vi "Teleop.vi"(10 "Match Info":T1={"Autonomous Elapsed Seconds"=0.0, "TeleOp Elapsed Seconds"=0.0, "Disabled Elapsed Seconds"=0.0, "Visited Autonomous"=FALSE, "Visited TeleOp"=FALSE, "Visited Disabled"=FALSE, "Autonomous Settings"={"Autonomous Style"=enum."Independent", "VI Refnum"=refnum}}, 11 "Call Context":T2) -> ()   [LabVIEW 2015]
doc: "This VI is called for each TeleOp packet received from the DS where the robot is not disabled. It is often used to read from the joysticks and update I/O or to update setpoints for timed control loops. It should complete and return within 20 milliseconds or it may miss DS packets."
uses:
  <vilib>/Rock Robotics/WPI/DriverStation/WPI_DriverStationDerivedRobotMode.ctl
  <vilib>/Rock Robotics/WPI/DriverStation/WPI_DriverStationMatch Info.ctl
  <vilib>/Rock Robotics/WPI/Solenoid/WPI_SolenoidValue.ctl
  <vilib>/Rock Robotics/WPI/Utilities/WPI_GetSetVariantRefNum.vi
  <vilib>/Rock Robotics/Network Tables/NT Write Boolean Array.vi
  <vilib>/Rock Robotics/Network Tables/NT Write Numeric Array.vi
  <vilib>/Rock Robotics/Network Tables/NT Read Boolean.vi
  <vilib>/Rock Robotics/Network Tables/NT Read Number.vi
  <vilib>/Rock Robotics/WPI/Solenoid/WPI_SolenoidSetEnum.vi
  <vilib>/Rock Robotics/Network Tables/NT Write Boolean.vi
  <vilib>/addons/control/pid/NI_PID_pid.lvlib
  <vilib>/addons/control/pid/pid.llb/PID (DBL).vi
panel:
  out "Angle":dbl
  out "Distance":dbl
  out "Sample Slider 0":dbl(slide) scale=0.0..5.0
  out "Sample Boolean 1":bool
  out "Sample Boolean 0":bool
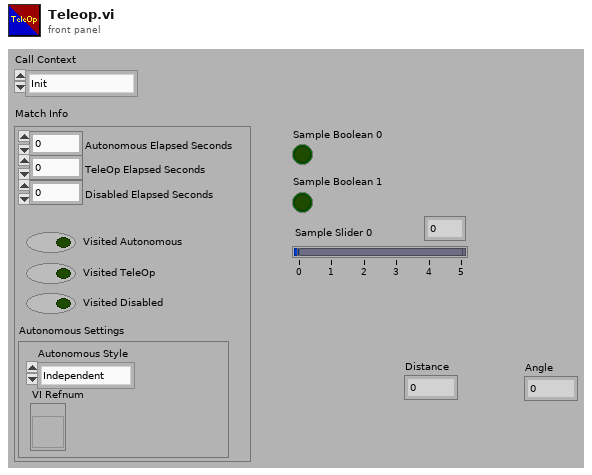
[diagram p1: front panel]
types:
  T1 = typedef "WPI_DriverStationMatch Info.ctl" = cluster{"Autonomous Elapsed Seconds":dbl, "TeleOp Elapsed Seconds":dbl, "Disabled Elapsed Seconds":dbl, "Visited Autonomous":bool, "Visited TeleOp":bool, "Visited Disabled":bool, "Autonomous Settings":cluster{"Autonomous Style":enum16{"Iterative", "Independent"}, "VI Refnum":refnum<vi>}}
  T2 = typedef "WPI_DriverStationDerivedRobotMode.ctl" = enum16{"Init", "Execute", "Stop"}
  T3 = typedef "WPI_SolenoidValue.ctl" = enum16{"Off", "On", "Forward", "Reverse"}
  T4 = typedef "WPI_AnalogChannelDevRef.ctl" = cluster{"DevStatus":errorcluster, "Analog Channel":T5}
  T5 = typedef "FPGA_AIChannel.ctl" = enum8{"AI 0", "AI 1", "AI 2", "AI 3", "AI MXP 0", "AI MXP 1", "AI MXP 2", "AI MXP 3", "Invalid"}
  T6 = typedef "WPI_JoystickDevRef.ctl" = cluster{"Device":T7}
  T7 = typedef "WPI_JoystickDeviceEnum.ctl" = enum16{"USB 0", "USB 1", "USB 2", "USB 3", "USB 4", "USB 5"}
  T8 = cluster{"Buttons[0]":bool, "Buttons[1]":bool, "Buttons[2]":bool, "Buttons[3]":bool, "Buttons[4]":bool, "Buttons[5]":bool, "Buttons[6]":bool, "Buttons[7]":bool, "Buttons[8]":bool}
  T9 = typedef "WPI_MotorControlDeviceRef.ctl" = cluster{"DeviceStatus":errorcluster, "Type":T10, "PWM":cluster{"PWM Channel":T11, "DeadBand":T12}, "CAN":cluster{"Device Number":u8, "Control Mode":T13, "Semaphore":T14, "Max Vout":dbl, "TalonSRX Control Mode":T15}, "Invert":bool}
  T10 = typedef "WPI_MotorControlType.ctl" = enum16{"PWM", "CAN", "CANTalonSRX"}
  T11 = typedef "FPGA_DIOPWMChannel.ctl" = enum8{"PWM 0", "PWM 1", "PWM 2", "PWM 3", "PWM 4", "PWM 5", "PWM 6", "PWM 7", "PWM 8", "PWM 9", "PWM MXP 0", "PWM MXP 1", "PWM MXP 2", "PWM MXP 3", "PWM MXP 4", "PWM MXP 5", "PWM MXP 6", "PWM MXP 7", "PWM MXP 8", "PWM MXP 9", "Invalid"}
  T12 = typedef "WPI_PWMDeadband.ctl" = cluster{"Name":string, "maxPositivePwm":i32, "minPositivePwm":i32, "centerPwm":i32, "maxNegativePwm":i32, "minNegativePwm":i32, "angularRange":u16}
  T13 = typedef "WPI_CANJaguar_ControlMode.ctl" = enum8{"Percent VBus", "Current", "Speed", "Position", "Voltage"}
  T14 = typedef "Semaphore RefNum" = refnum<k1>
  T15 = typedef "WPI_CANTalonSRX_APIControlMode.ctl" = enum8{"Percent VBus", "Speed", "Position", "Slave", "Unchanged / Invalid", "Voltage Compensation", "Current", "Motion Profile"}
  T16 = cluster{"proportional gain (Kc)":dbl, "integral time (Ti, min)":dbl, "derivative time (Td, min)":dbl}
  T17 = typedef "WPI_RobotDriveDevRef.ctl" = cluster{"DevStatus":errorcluster, "Motors[]":T9[], "Square Inputs":bool, "Max Output":dbl}
  T18 = typedef "WPI_SolenoidDevRef.ctl" = cluster{"DevStatus":errorcluster, "Pneumatics Control Module":u8, "Forward Solenoid Channel":T19, "Reverse Solenoid Channel":T19}
  T19 = typedef "WPI_SolenoidChannel.ctl" = enum8{"Solenoid 0", "Solenoid 1", "Solenoid 2", "Solenoid 3", "Solenoid 4", "Solenoid 5", "Solenoid 6", "Solenoid 7", "Invalid"}
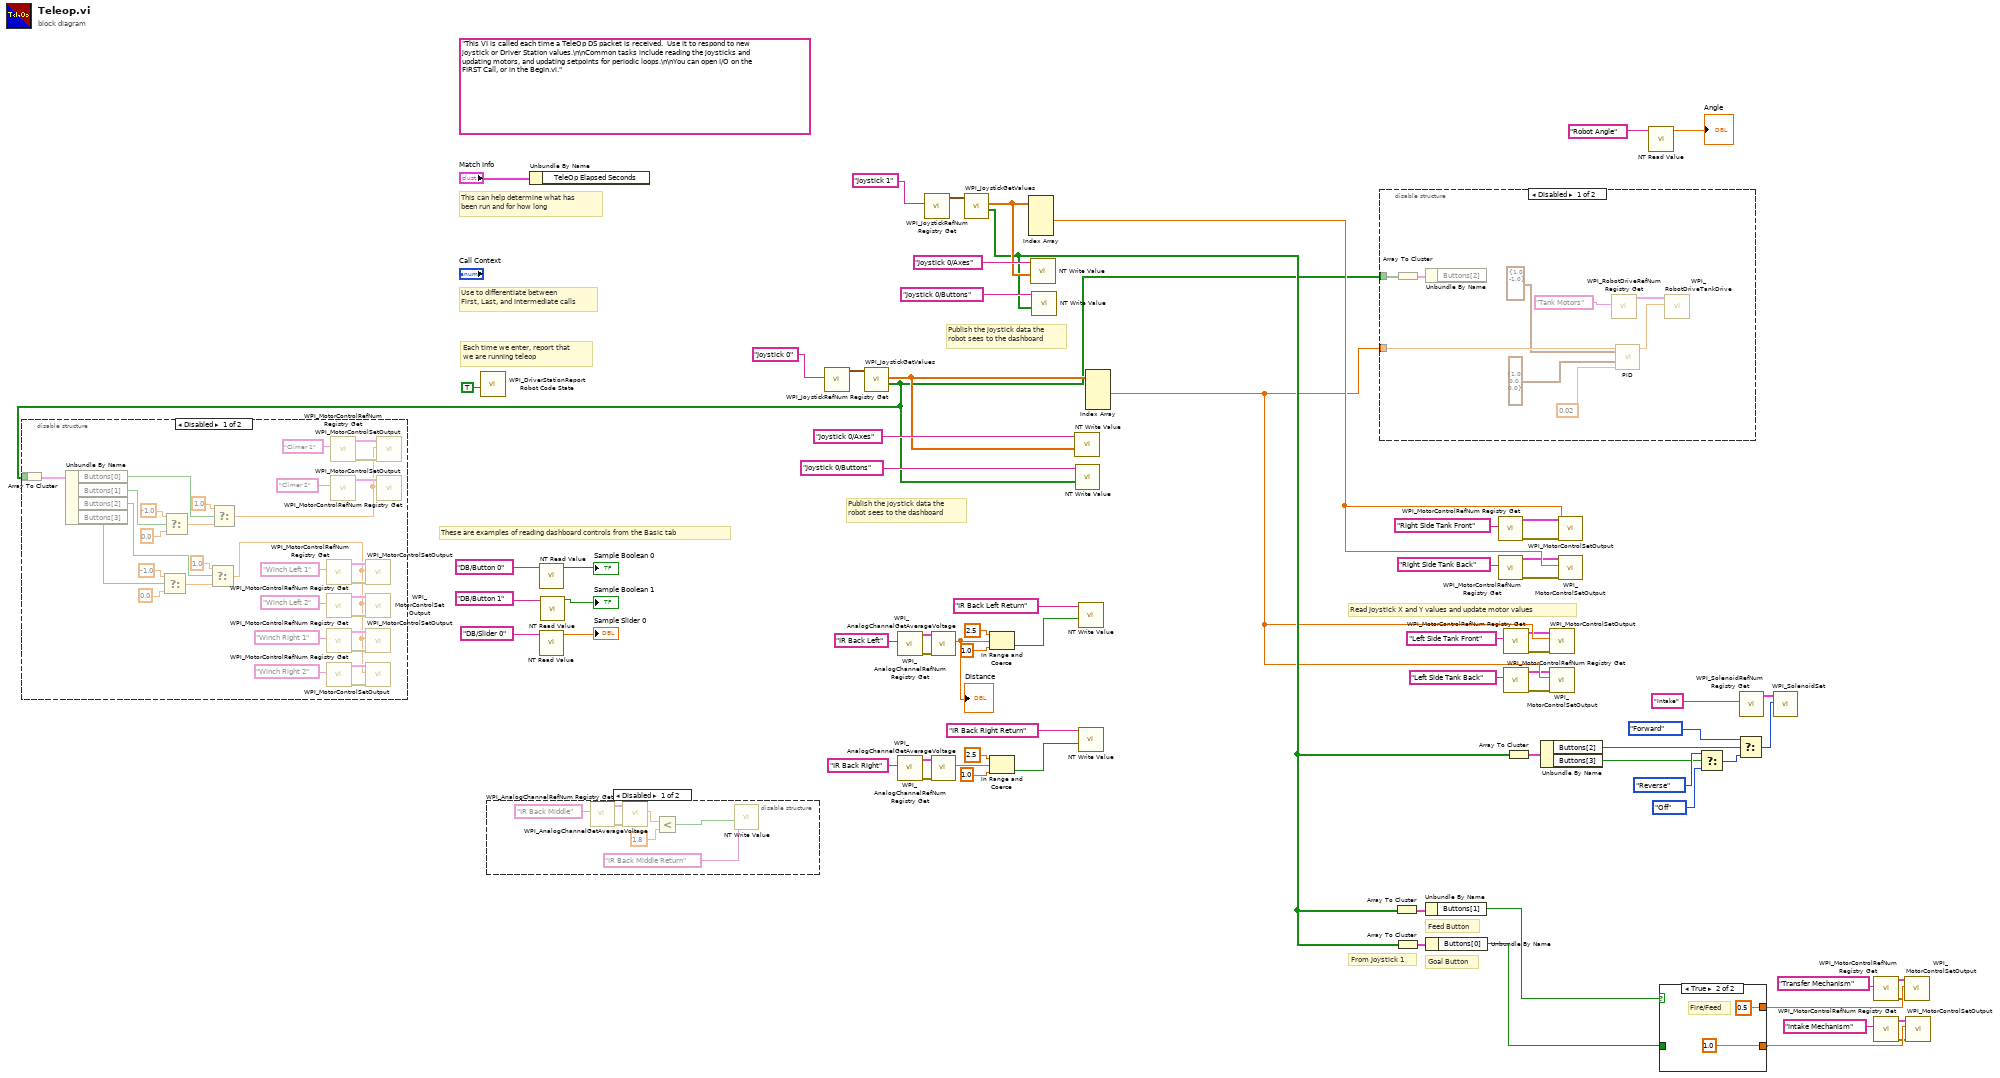
[diagram p0: block diagram]
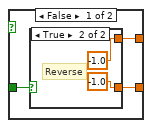
[diagram p5: hidden frame]
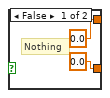
[diagram p6: hidden frame]
diagram:
  (unwired) "This VI is called each time a TeleOp DS packet is received.  Use it to respond to new joystick or Driver Station values.\n\nCommon tasks include reading the joysticks and updating motors, and updating setpoints for periodic loops.\n\nYou can open I/O on the FIRST Call, or in the Begin.vi."
  # "Read Joystick X and Y values and update motor values"
  # "From Joystick 1"
  # "Feed Button"
  # "Goal Button"
  # "Publish the joystick data the\nrobot sees to the dashboard"
  # "These are examples of reading dashboard controls from the Basic tab"
  # "Publish the joystick data the\nrobot sees to the dashboard"
  # "Each time we enter, report that\nwe are running teleop"
  # "Use to differentiate between\nFirst, Last, and Intermediate calls"
  # "This can help determine what has\nbeen run and for how long"
  n1 = call <vilib>:"WPI_DriverStationReport Robot Code State.vi"("TeleOp"=TRUE ("Autonomous")) -> ()  [unwired: 10 in, 1 out]
  n2 = disable-structure shown="Disabled" {
    frame Disabled {
      n3 = call <vilib>:"WPI_AnalogChannelRefNum Registry Get.vi"("refnum name"="IR Back Middle") -> ("error out"=w79:errorcluster, "AIDeviceRef"=w80:T4)  [unwired: 9 in]
      n4 = call <vilib>:"WPI_AnalogChannelGetAverageVoltage.vi"("error in (no error)"=w79, "AIDeviceRef"=w80) -> ("Voltage"=w78:dbl)  [unwired: 7 in, 2 out]
      n5 = Less?(x=w78, y=1.8) -> (x < y?=w76:bool)
      n6 = call-poly <vilib>:"NT Write Value.vi"("Boolean"=w76, "Name"="IR Back Middle Return") -> ()  [unwired: 9 in, 1 out]
    }
    frame Enabled {
    }
  }
  n7 = Unbundle By Name("Match Info") -> ()  [unwired: 1 out]
  n8 = call-poly <vilib>:"NT Read Value.vi"("Name"="DB/Button 0" ("refnum name")) -> ("Boolean"=→"Sample Boolean 0":bool)  [unwired: 9 in, 1 out]
  n9 = call-poly <vilib>:"NT Read Value.vi"("Name"="DB/Slider 0" ("refnum name")) -> ("Numeric"=→"Sample Slider 0":dbl)  [unwired: 9 in, 1 out]
  n10 = call-poly <vilib>:"NT Read Value.vi"("Name"="DB/Button 1" ("refnum name")) -> ("Boolean"=→"Sample Boolean 1":bool)  [unwired: 9 in, 1 out]
  n11 = call <vilib>:"WPI_JoystickRefNum Registry Get.vi"("refnum name"="Joystick 0") -> ("JoystickDevRef"=w72:T6)  [unwired: 1 in, 9 out]
  n12 = call <vilib>:"WPI_JoystickGetValues.vi"("JoystickDevRef"=w72) -> ("Buttons"=w3:bool[], "Axes"=w68:dbl[])  [unwired: 6 in, 3 out]
  n13 = disable-structure shown="Disabled" {
    disable-tunnel: w3 -> [w114 _]
    frame Disabled {
      n14 = Array To Cluster(array=w114) -> (cluster=w113:T8)
      n15 = Unbundle By Name(w113) -> ("Buttons[0]"=w106:bool, "Buttons[1]"=w101:bool, "Buttons[2]"=w84:bool, "Buttons[3]"=w83:bool)
      n16 = Select(t=-1.0, s=w83, f=0.0) -> (s? t:f=w87:dbl)
      n17 = Select(t=-1.0, s=w101, f=0.0) -> (s? t:f=w104:dbl)
      n18 = Select(t=1.0, s=w84, f=w87) -> (s? t:f=w85:dbl)
      n19 = Select(t=1.0, s=w106, f=w104) -> (s? t:f=w90:dbl)
      n20 = call <vilib>:"WPI_MotorControlRefNum Registry Get.vi"("refnum name"="Winch Left 1") -> ("error out"=w107:errorcluster, "MotorControlDevRef"=w108:T9)  [unwired: 9 in]
      n21 = call <vilib>:"WPI_MotorControlRefNum Registry Get.vi"("refnum name"="Winch Left 2") -> ("error out"=w99:errorcluster, "MotorControlDevRef"=w98:T9)  [unwired: 9 in]
      n22 = call <vilib>:"WPI_MotorControlRefNum Registry Get.vi"("refnum name"="Winch Right 1") -> ("error out"=w94:errorcluster, "MotorControlDevRef"=w95:T9)  [unwired: 9 in]
      n23 = call <vilib>:"WPI_MotorControlRefNum Registry Get.vi"("refnum name"="Winch Right 2") -> ("error out"=w93:errorcluster, "MotorControlDevRef"=w92:T9)  [unwired: 9 in]
      n24 = call <vilib>:"WPI_MotorControlRefNum Registry Get.vi"("refnum name"="Climer 1") -> ("error out"=w110:errorcluster, "MotorControlDevRef"=w111:T9)  [unwired: 9 in]
      n25 = call <vilib>:"WPI_MotorControlRefNum Registry Get.vi"("refnum name"="Climer 2") -> ("MotorControlDevRef"=w100:T9)  [unwired: 9 in, 1 out]
      n26 = call <vilib>:"WPI_MotorControlSetOutput.vi"("error in (no error)"=w107, "Output"=w85, "MotorControlDevRef"=w108) -> ()  [unwired: 6 in, 3 out]
      n27 = call <vilib>:"WPI_MotorControlSetOutput.vi"("error in (no error)"=w99, "Output"=w85, "MotorControlDevRef"=w98) -> ()  [unwired: 6 in, 3 out]
      n28 = call <vilib>:"WPI_MotorControlSetOutput.vi"("error in (no error)"=w94, "Output"=w85, "MotorControlDevRef"=w95) -> ()  [unwired: 6 in, 3 out]
      n29 = call <vilib>:"WPI_MotorControlSetOutput.vi"("error in (no error)"=w93, "Output"=w85, "MotorControlDevRef"=w92) -> ()  [unwired: 6 in, 3 out]
      n30 = call <vilib>:"WPI_MotorControlSetOutput.vi"("error in (no error)"=w110, "Output"=w90, "MotorControlDevRef"=w111) -> ()  [unwired: 6 in, 3 out]
      n31 = call <vilib>:"WPI_MotorControlSetOutput.vi"("Output"=w90, "MotorControlDevRef"=w100) -> ()  [unwired: 7 in, 3 out]
    }
    frame Enabled {
    }
  }
  n32 = call <vilib>:"WPI_AnalogChannelRefNum Registry Get.vi"("refnum name"="IR Back Left") -> ("error out"=w35:errorcluster, "AIDeviceRef"=w36:T4)  [unwired: 9 in]
  n33 = call <vilib>:"WPI_AnalogChannelRefNum Registry Get.vi"("refnum name"="IR Back Right") -> ("error out"=w25:errorcluster, "AIDeviceRef"=w24:T4)  [unwired: 9 in]
  n34 = call <vilib>:"WPI_JoystickRefNum Registry Get.vi"("refnum name"="Joystick 1") -> ("JoystickDevRef"=w60:T6)  [unwired: 1 in, 9 out]
  n35 = call <vilib>:"WPI_AnalogChannelGetAverageVoltage.vi"("error in (no error)"=w35, "AIDeviceRef"=w36) -> ("Voltage"=w27:dbl)  [unwired: 7 in, 2 out]
  "Distance" <- w27
  n36 = call <vilib>:"WPI_AnalogChannelGetAverageVoltage.vi"("error in (no error)"=w25, "AIDeviceRef"=w24) -> ("Voltage"=w19:dbl)  [unwired: 7 in, 2 out]
  n37 = call <vilib>:"WPI_JoystickGetValues.vi"("JoystickDevRef"=w60) -> ("Buttons"=w33:bool[], "Axes"=w38:dbl[])  [unwired: 6 in, 3 out]
  n38 = In Range and Coerce(upper limit=2.5, x=w27, lower limit=1.0) -> (In Range?=w26:bool)  [unwired: 1 out]
  n39 = In Range and Coerce(upper limit=2.5, x=w19, lower limit=1.0) -> (In Range?=w18:bool)  [unwired: 1 out]
  n40 = Index Array(array=w38) -> (element #2=w17:dbl)  [unwired: 4 in, 3 out]
  n41 = call-poly <vilib>:"NT Write Value.vi"("Numeric Array"=w38, "Name"="Joystick 0/Axes") -> ()  [unwired: 9 in, 1 out]
  n42 = call-poly <vilib>:"NT Write Value.vi"("Boolean Array"=w33, "Name"="Joystick 0/Buttons") -> ()  [unwired: 9 in, 1 out]
  n43 = call-poly <vilib>:"NT Write Value.vi"("Numeric Array"=w68, "Name"="Joystick 0/Axes") -> ()  [unwired: 9 in, 1 out]
  n44 = call-poly <vilib>:"NT Write Value.vi"("Boolean Array"=w3, "Name"="Joystick 0/Buttons") -> ()  [unwired: 9 in, 1 out]
  n45 = call-poly <vilib>:"NT Write Value.vi"("Boolean"=w26, "Name"="IR Back Left Return") -> ()  [unwired: 9 in, 1 out]
  n46 = call-poly <vilib>:"NT Write Value.vi"("Boolean"=w18, "Name"="IR Back Right Return") -> ()  [unwired: 9 in, 1 out]
  n47 = Index Array(array=w68) -> (element #2=w16:dbl)  [unwired: 4 in, 3 out]
  n48 = disable-structure shown="Disabled" {
    disable-tunnel: w16 -> [w120 _]
    disable-tunnel: w3 -> [w115 _]
    frame Disabled {
      n49 = Array To Cluster(array=w115) -> (cluster=w116:T8)
      n50 = Unbundle By Name(w116) -> ()  [unwired: 1 out]
      n51 = call <vilib>:"WPI_RobotDriveRefNum Registry Get.vi"("refnum name"="Tank Motors") -> ("RobotDriveDevRef"=w122:T17)  [unwired: 9 in, 1 out]
      n52 = call-poly <vilib>:"PID.vi"("output range"=cluster{"output high":dbl, "output low":dbl} {"output high"=1.0, "output low"=-1.0}, "dt (s)"=0.02, "PID gains"=T16 {"proportional gain (Kc)"=1.0, "integral time (Ti, min)"=0.0, "derivative time (Td, min)"=0.0}, "setpoint"=w120) -> ("output"=w121:dbl)  [unwired: 6 in, 1 out]
      n53 = call <vilib>:"WPI_RobotDriveTankDrive.vi"("Left axis value"=w121, "RobotDriveDevRef"=w122) -> ()  [unwired: 7 in, 3 out]
    }
    frame Enabled {
    }
  }
  n54 = Array To Cluster(array=w33) -> (cluster=w32:T8)
  n55 = Array To Cluster(array=w33) -> (cluster=w39:T8)
  n56 = Unbundle By Name(w32) -> ("Buttons[1]"=w31:bool)
  n57 = Unbundle By Name(w39) -> ("Buttons[0]"=w30:bool)
  n58 = call <vilib>:"WPI_MotorControlRefNum Registry Get.vi"("refnum name"="Right Side Tank Front") -> ("error out"=w7:errorcluster, "MotorControlDevRef"=w8:T9)  [unwired: 9 in]
  n59 = call <vilib>:"WPI_MotorControlRefNum Registry Get.vi"("refnum name"="Right Side Tank Back") -> ("error out"=w4:errorcluster, "MotorControlDevRef"=w5:T9)  [unwired: 9 in]
  n60 = call <vilib>:"WPI_MotorControlRefNum Registry Get.vi"("refnum name"="Left Side Tank Front") -> ("error out"=w13:errorcluster, "MotorControlDevRef"=w14:T9)  [unwired: 9 in]
  n61 = call <vilib>:"WPI_MotorControlRefNum Registry Get.vi"("refnum name"="Left Side Tank Back") -> ("error out"=w10:errorcluster, "MotorControlDevRef"=w11:T9)  [unwired: 9 in]
  n62 = Array To Cluster(array=w33) -> (cluster=w50:T8)
  n63 = Unbundle By Name(w50) -> ("Buttons[2]"=w49:bool, "Buttons[3]"=w48:bool)
  n64 = call <vilib>:"WPI_MotorControlSetOutput.vi"("error in (no error)"=w13, "Output"=w16, "MotorControlDevRef"=w14) -> ()  [unwired: 6 in, 3 out]
  n65 = call <vilib>:"WPI_MotorControlSetOutput.vi"("error in (no error)"=w10, "Output"=w16, "MotorControlDevRef"=w11) -> ()  [unwired: 6 in, 3 out]
  n66 = call <vilib>:"WPI_MotorControlSetOutput.vi"("error in (no error)"=w7, "Output"=w17, "MotorControlDevRef"=w8) -> ()  [unwired: 6 in, 3 out]
  n67 = call <vilib>:"WPI_MotorControlSetOutput.vi"("error in (no error)"=w4, "Output"=w17, "MotorControlDevRef"=w5) -> ()  [unwired: 6 in, 3 out]
  n68 = call-poly <vilib>:"NT Read Value.vi"("Name"="Robot Angle") -> ("Numeric"=→"Angle":dbl)  [unwired: 9 in, 1 out]
  n69 = case shown="True" w31 {
    tunnel: [w126 0.5] -> w47
    tunnel: [w125 1.0] -> w46
    tunnel: w30 -> [w124 _]
    frame False {
      n70 = case shown="True" w124 {
        tunnel: [0.0 -1.0] -> w126
        tunnel: [0.0 -1.0] -> w125
        frame False {
          # "Nothing"
        }
        frame True {
          # "Reverse"
        }
      }
    }
    frame True {
      # "Fire/Feed"
    }
  }
  n71 = Select(t=WPI_SolenoidValue."Reverse" ("Value"), s=w48, f=WPI_SolenoidValue."Off") -> (s? t:f=w51:T3)
  n72 = Select(t=WPI_SolenoidValue."Forward" ("Value"), s=w49, f=w51) -> (s? t:f=w55:T3)
  n73 = call <vilib>:"WPI_SolenoidRefNum Registry Get.vi"("refnum name"="Intake") -> ("SolenoidDevRef"=w54:T18)  [unwired: 9 in, 1 out]
  n74 = call-poly <vilib>:"WPI_SolenoidSet.vi"("Value"=w55, "SolenoidDevRef"=w54) -> ()  [unwired: 1 in, 9 out]
  n75 = call <vilib>:"WPI_MotorControlRefNum Registry Get.vi"("refnum name"="Transfer Mechanism") -> ("error out"=w42:errorcluster, "MotorControlDevRef"=w40:T9)  [unwired: 9 in]
  n76 = call <vilib>:"WPI_MotorControlRefNum Registry Get.vi"("refnum name"="Intake Mechanism") -> ("error out"=w45:errorcluster, "MotorControlDevRef"=w44:T9)  [unwired: 9 in]
  n77 = call <vilib>:"WPI_MotorControlSetOutput.vi"("error in (no error)"=w42, "Output"=w47, "MotorControlDevRef"=w40) -> ()  [unwired: 6 in, 3 out]
  n78 = call <vilib>:"WPI_MotorControlSetOutput.vi"("error in (no error)"=w45, "Output"=w46, "MotorControlDevRef"=w44) -> ()  [unwired: 6 in, 3 out]
